vi "Set Sensor Params by Index.vi"(9 "Index":i32, 11 "Sensor Cfg Params":T1={"Total Pixels"=0, "Positive  Peaks"=FALSE, "CalibrCoefArray"=[0.0, 0.0, 0.0, 0.0, 0.0], "Start Idx"=0, "End Idx"=0} {"CalibrCoefArray" format="%#.12g"}) -> ()   [LabVIEW 2015, in "Tool Cfg.lvlib"]
uses:
  Tool Cfg.lvlib
  _SensorConfigParams Cluster--typedef.ctl
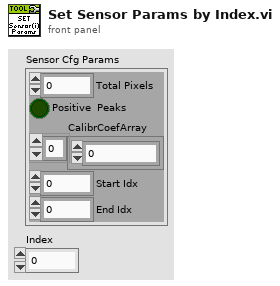
[diagram p1: front panel]
types:
  T1 = typedef "Tool Cfg.lvlib/_SensorConfigParams Cluster--typedef.ctl" = cluster{"Total Pixels":u16, "Positive  Peaks":bool, "CalibrCoefArray":dbl[], "Start Idx":u16, "End Idx":u16}
  T2 = typedef "Tool Cfg.lvlib/_ProbeConfigParams Cluster--typedef.ctl" = cluster{"Name":string, "Laser Init Pwr":u16, "Laser Gain":u8, "Integ Count":u16, "Meas. Range":sgl, "Angle":sgl, "Probe Offset":sgl, "Sensor Block":T3}
  T3 = typedef "Tool Cfg.lvlib/_Sensor Block Cluster--typedef.ctl" = cluster{"nSensors":u16, "SensorCfgParams Array":T1[]}
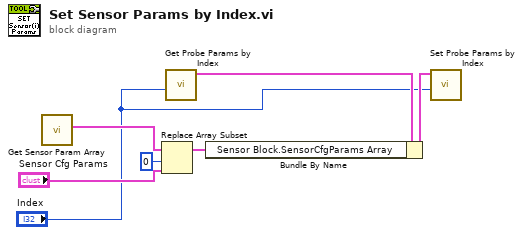
[diagram p0: block diagram]
diagram:
  n1 = call "Get Sensor Param Array.vi"() -> ("Sensor Block.SensorCfgParams Array"=w7:T1[])  [unwired: 10 in, 1 out]
  n2 = Replace Array Subset(array=w7, new element="Sensor Cfg Params", index=0) -> (w3:T1[])
  n3 = call "Get Probe Params by Index.vi"("Probe Select"="Index") -> ("Probe Cfg Params"=w4:T2)  [unwired: 10 in]
  n4 = Bundle By Name(cluster=w4, "Sensor Block.SensorCfgParams Array"=w3) -> (w2:T2)
  n5 = call "Set Probe Params by Index.vi"("Index"="Index", "Probe Cfg Params"=w2) -> ()  [unwired: 10 in]
